vi "svInitSerial.vi"(8 "error in":errorcluster, 11 "VISA Refnum in":refnum<visa-resource-name>) -> (0 "error out":errorcluster, 3 "VISA Refnum out":refnum<visa-resource-name>)   [LabVIEW 2022 SP3]
uses:
  <vilib>/Instr/_visa.llb/VISA Configure Serial Port (Instr).vi
  Serial - Settings.ctl
  Serial - ASCII Characters.ctl
  Serial - XON-XOFF Characters.ctl
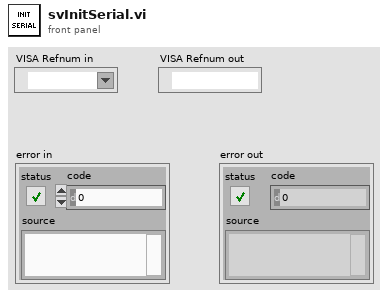
[diagram p1: front panel]
types:
  T1 = typedef "Serial - XON-XOFF Characters.ctl" = cluster{"XON":T2, "XOFF":T2}
  T2 = typedef "Serial - ASCII Characters.ctl" = enum16{"NUL", "SOH", "STX", "ETX", "EOT", "ENQ", "ACK", "BEL", "BS", "HT", "LF", "VT", "FF", "CR", "SO", "SI", "DLE", "DC1", "DC2", "DC3", "DC4", "NAK", "SYN", "ETB", "CAN", "EM", "SUB", "ESC", "FS", "GS", "RS", "US", "SP", "!", "\"", "#", "$", "%", "&", "'", "(", ")", "*", "+", ",", "- (-)", ".", "/", "0", "1", "2", "3", "4", "5", "6", "7", "8", "9", ":", ";", "<", "=", ">", "?", "@", "A", "B", "C", "D", "E", "F", "G", "H", "I", "J", "K", "L", "M", "N", "O", "P", "Q", "R", "S", "T", "U", "V", "W", "X", "Y", "Z", "[", "\\", "]", "^", "_", "`", "a", "b", "c", "d", "e", "f", "g", "h", "i", "j", "k", "l", "m", "n", "o", "p", "q", "r", "s", "t", "u", "v", "w", "x", "y", "z", "{", "|", "}", "~"}
  T3 = typedef "Serial - Settings.ctl" = cluster{"baud rate":u32, "data bits":u16, "parity":enum16{"None", "Odd", "Even", "Mark", "Space"}, "stop bits":u16, "flow control":u16}
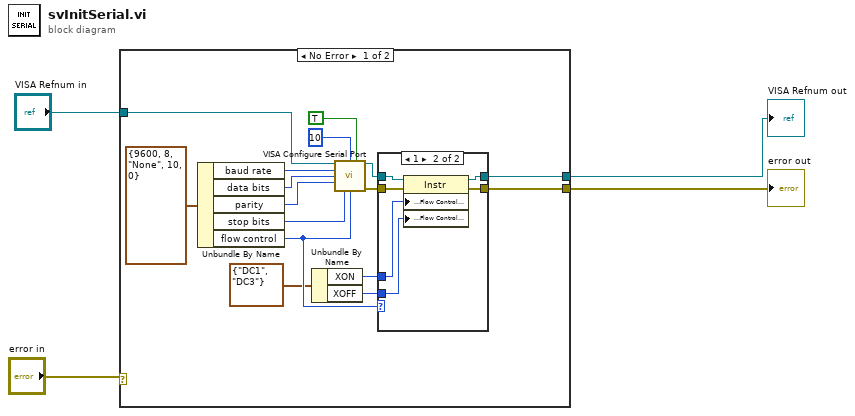
[diagram p0: block diagram]
diagram:
  n1 = case shown="No Error" "error in" {
    selector: "error in" -> [_ w30]
    tunnel: [w19 w29] -> w4
    tunnel: [w18 w30] -> w3
    tunnel: "VISA Refnum in" -> [w5 w29]
    frame No Error {
      n2 = Unbundle By Name(T3 {"baud rate"=9600, "data bits"=8, "parity"=enum."None", "stop bits"=10, "flow control"=0} ("Serial Settings")) -> ("baud rate"=w12:u32, "data bits"=w11:u16, "parity"=w10:enum16{"None", "Odd", "Even", "Mark", "Space"}, "stop bits"=w9:u16, "flow control"=w15:u16)
      n3 = Unbundle By Name(T1 {"XON"=enum."DC1", "XOFF"=enum."DC3"} ("XON/XOFF Characters")) -> ("XON"=w16:T2, "XOFF"=w17:T2)
      n4 = call-poly "VISA Configure Serial Port"("VISA resource name"=w5, "termination char\n(0xA = '\\n' = LF)"=u8 10 ("Termination Character"), "Enable Termination\nChar (T)"=TRUE ("End Read on Termination Character?"), "baud rate (9600)"=w12, "data bits (8)"=w11, "parity (0:none)"=w10, "stop bits (10: 1 bit)"=w9, "flow control (0:none)"=w15) -> ("VISA resource name out"=w8:refnum<visa-resource-name>, "error out"=w7:errorcluster)  [unwired: 2 in, 4 out]
      n5 = case shown="1" w15 {
        tunnel: [w21 w28] -> w18
        tunnel: [w22 w27] -> w19
        tunnel: w7 -> [w21 w26]
        tunnel: w8 -> [w22 w25]
        tunnel: w16 -> [_ w24]
        tunnel: w17 -> [_ w23]
        frame Default {
        }
        frame 1 {
          n6 = property class="Instr"(reference=w25, error in=w26, "Serial Settings:Flow Control XON Character"=w24, "Serial Settings:Flow Control XOFF Character"=w23) -> (reference out=w27:refnum<visa-resource-name>, error out=w28:errorcluster)
        }
      }
    }
    frame Error {
    }
  }
  "VISA Refnum out" <- w4
  "error out" <- w3
